vi "test OpenScalar.vi"(8 "error in (no error)":errorcluster) -> (0 "error out":errorcluster)   [LabVIEW 2020]
uses:
  <vilib>/addons/_JKI Toolkits/Caraya/classes/Test/Test.lvclass
  <vilib>/addons/_JKI Toolkits/Caraya/classes/Assert/Assert.lvclass
  _built_ppls/OpenScalar.lvlibp
  <vilib>/addons/_JKI Toolkits/Caraya/classes/Assert/Assert Equal Value and Type_Variant.vi
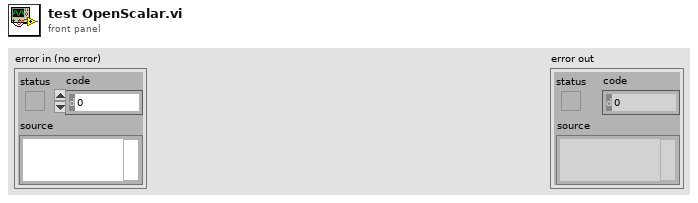
[diagram p1: front panel]
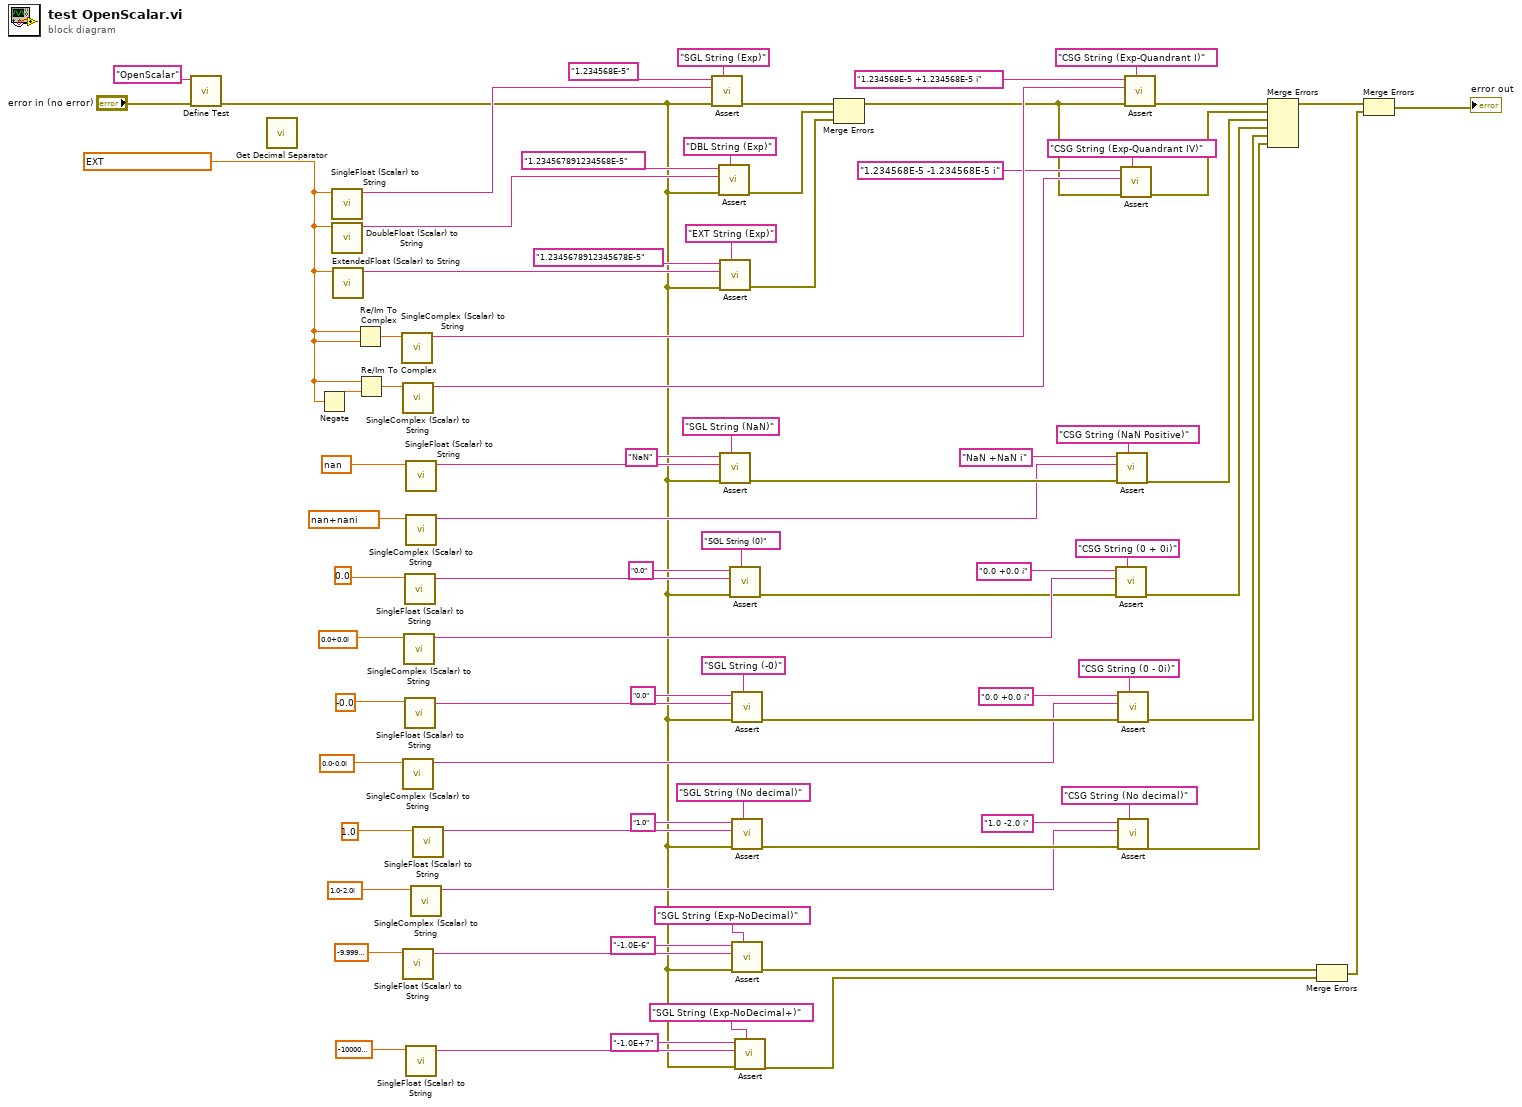
[diagram p0: block diagram]
diagram:
  w59 = ext 0.000012345678912345678
  n1 = call <vilib>:"Define Test.vi"("error in (no error)"="error in (no error)", "Label (VI Title)"="OpenScalar") -> ("error out"=w2:errorcluster)  [unwired: 8 in, 1 out]
  n2 = call "Get Decimal Separator.vi"() -> ()  [unwired: 11 in, 1 out]
  n3 = Negate(x=w59) -> (-x=w75:ext)
  n4 = call "SingleFloat (Scalar) to String.vi"("Value (Single)"=w59) -> ("Value (String)"=w74:string)  [unwired: 10 in]
  n5 = call "DoubleFloat (Scalar) to String.vi"("Value (Double)"=w59) -> ("Value (String)"=w70:string)  [unwired: 10 in]
  n6 = call "ExtendedFloat (Scalar) to String.vi"("Value (Extended)"=w59) -> ("Value (String)"=w65:string)  [unwired: 10 in]
  n7 = Re/Im To Complex(1:w59, 2:w59) -> (0:w77:cxt)
  n8 = Re/Im To Complex(1:w75, 2:w59) -> (0:w76:cxt)
  n9 = call "SingleComplex (Scalar) to String.vi"("Value (CSG)"=w77) -> ("Value (String)"=w58:string)  [unwired: 10 in]
  n10 = call "SingleComplex (Scalar) to String.vi"("Value (CSG)"=w76) -> ("Value (String)"=w54:string)  [unwired: 10 in]
  n11 = call "SingleComplex (Scalar) to String.vi"("Value (CSG)"=csg 0.0-0.0i) -> ("Value (String)"=w26:string)  [unwired: 10 in]
  n12 = call "SingleFloat (Scalar) to String.vi"("Value (Single)"=sgl -1e-06) -> ("Value (String)"=w10:string)  [unwired: 10 in]
  n13 = call "SingleComplex (Scalar) to String.vi"("Value (CSG)"=csg 0.0+0.0i) -> ("Value (String)"=w38:string)  [unwired: 10 in]
  n14 = call "SingleFloat (Scalar) to String.vi"("Value (Single)"=sgl 0.0) -> ("Value (String)"=w33:string)  [unwired: 10 in]
  n15 = call "SingleFloat (Scalar) to String.vi"("Value (Single)"=sgl -0.0) -> ("Value (String)"=w24:string)  [unwired: 10 in]
  n16 = call "SingleFloat (Scalar) to String.vi"("Value (Single)"=sgl nan) -> ("Value (String)"=w45:string)  [unwired: 10 in]
  n17 = call "SingleComplex (Scalar) to String.vi"("Value (CSG)"=csg nan+nani) -> ("Value (String)"=w39:string)  [unwired: 10 in]
  n18 = call "SingleFloat (Scalar) to String.vi"("Value (Single)"=sgl -10000000.0) -> ("Value (String)"=w6:string)  [unwired: 10 in]
  n19 = call "SingleComplex (Scalar) to String.vi"("Value (CSG)"=csg 1.0-2.0i) -> ("Value (String)"=w15:string)  [unwired: 10 in]
  n20 = call "SingleFloat (Scalar) to String.vi"("Value (Single)"=sgl 1.0) -> ("Value (String)"=w14:string)  [unwired: 10 in]
  n21 = call-poly <vilib>:"Assert.vi"("Label"="SGL String (Exp)" ("Label (VI Title)"), "error in (no error)"=w2, "Y"=w74, "X"="1.234568E-5" ("Label (VI Title)")) -> ("error out"=w68:errorcluster)  [unwired: 6 in, 1 out]
  n22 = call-poly <vilib>:"Assert.vi"("Label"="DBL String (Exp)" ("Label (VI Title)"), "error in (no error)"=w2, "Y"=w70, "X"="1.234567891234568E-5" ("Label (VI Title)")) -> ("error out"=w69:errorcluster)  [unwired: 6 in, 1 out]
  n23 = call-poly <vilib>:"Assert.vi"("Label"="EXT String (Exp)" ("Label (VI Title)"), "error in (no error)"=w2, "Y"=w65, "X"="1.2345678912345678E-5" ("Label (VI Title)")) -> ("error out"=w66:errorcluster)  [unwired: 6 in, 1 out]
  n24 = call-poly <vilib>:"Assert.vi"("Label"="SGL String (NaN)" ("Label (VI Title)"), "error in (no error)"=w2, "Y"=w45, "X"="NaN" ("Label (VI Title)")) -> ("error out"=w44:errorcluster)  [unwired: 6 in, 1 out]
  n25 = call-poly <vilib>:"Assert.vi"("Label"="SGL String (0)" ("Label (VI Title)"), "error in (no error)"=w2, "Y"=w33, "X"="0.0" ("Label (VI Title)")) -> ("error out"=w31:errorcluster)  [unwired: 6 in, 1 out]
  n26 = call-poly <vilib>:"Assert.vi"("Label"="SGL String (-0)" ("Label (VI Title)"), "error in (no error)"=w2, "Y"=w24, "X"="0.0" ("Label (VI Title)")) -> ("error out"=w30:errorcluster)  [unwired: 6 in, 1 out]
  n27 = call-poly <vilib>:"Assert.vi"("Label"="SGL String (No decimal)" ("Label (VI Title)"), "error in (no error)"=w2, "Y"=w14, "X"="1.0" ("Label (VI Title)")) -> ("error out"=w18:errorcluster)  [unwired: 6 in, 1 out]
  n28 = call-poly <vilib>:"Assert.vi"("Label"="SGL String (Exp-NoDecimal)" ("Label (VI Title)"), "error in (no error)"=w2, "Y"=w10, "X"="-1.0E-6" ("Label (VI Title)")) -> ("error out"=w9:errorcluster)  [unwired: 6 in, 1 out]
  n29 = call-poly <vilib>:"Assert.vi"("Label"="SGL String (Exp-NoDecimal+)" ("Label (VI Title)"), "error in (no error)"=w2, "Y"=w6, "X"="-1.0E+7" ("Label (VI Title)")) -> ("error out"=w1:errorcluster)  [unwired: 6 in, 1 out]
  n30 = Merge Errors(w68, w69, w66) -> (w53:errorcluster)
  n31 = call-poly <vilib>:"Assert.vi"("Label"="CSG String (0 + 0i)" ("Label (VI Title)"), "error in (no error)"=w31, "Y"=w38, "X"="0.0 +0.0 i" ("Label (VI Title)")) -> ("error out"=w37:errorcluster)  [unwired: 6 in, 1 out]
  n32 = call-poly <vilib>:"Assert.vi"("Label"="CSG String (NaN Positive)" ("Label (VI Title)"), "error in (no error)"=w44, "Y"=w39, "X"="NaN +NaN i" ("Label (VI Title)")) -> ("error out"=w43:errorcluster)  [unwired: 6 in, 1 out]
  n33 = call-poly <vilib>:"Assert.vi"("Label"="CSG String (0 - 0i)" ("Label (VI Title)"), "error in (no error)"=w30, "Y"=w26, "X"="0.0 +0.0 i" ("Label (VI Title)")) -> ("error out"=w25:errorcluster)  [unwired: 6 in, 1 out]
  n34 = call-poly <vilib>:"Assert.vi"("Label"="CSG String (No decimal)" ("Label (VI Title)"), "error in (no error)"=w18, "Y"=w15, "X"="1.0 -2.0 i" ("Label (VI Title)")) -> ("error out"=w13:errorcluster)  [unwired: 6 in, 1 out]
  n35 = call-poly <vilib>:"Assert.vi"("Label"="CSG String (Exp-Quandrant IV)" ("Label (VI Title)"), "error in (no error)"=w53, "Y"=w54, "X"="1.234568E-5 -1.234568E-5 i" ("Label (VI Title)")) -> ("error out"=w56:errorcluster)  [unwired: 6 in, 1 out]
  n36 = call-poly <vilib>:"Assert.vi"("Label"="CSG String (Exp-Quandrant I)" ("Label (VI Title)"), "error in (no error)"=w53, "Y"=w58, "X"="1.234568E-5 +1.234568E-5 i" ("Label (VI Title)")) -> ("error out"=w63:errorcluster)  [unwired: 6 in, 1 out]
  n37 = Merge Errors(w63, w56, w43, w37, w25, w13) -> (w60:errorcluster)
  n38 = Merge Errors(w9, w1) -> (w8:errorcluster)
  n39 = Merge Errors(w60, w8) -> (→"error out":errorcluster)
